vi "Sequence Update.vi"(8 "error in (no error)":errorcluster, 10 "Sequence Record":T2, 11 "Connection Refnum":T1) -> (0 "error out":errorcluster, 3 "Connection Refnum":T1)   [LabVIEW 2011]
uses:
  Sequence Record.ctl
  SI.LIB/ODBC/SQL Controls/Connection Refnum.ctl
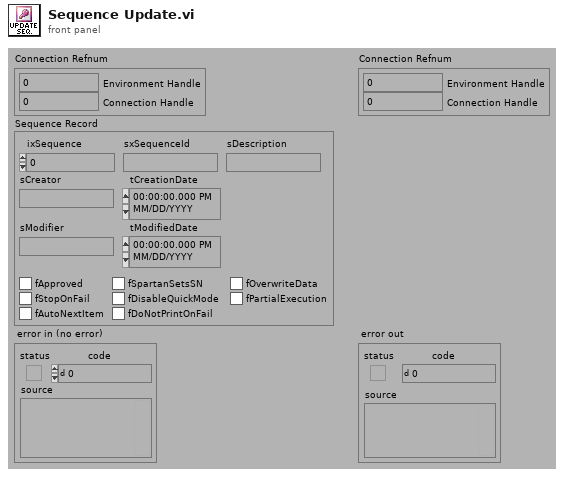
[diagram p1: front panel]
types:
  T1 = typedef "Connection Refnum.ctl" = cluster{"Environment Handle":i32, "Connection Handle":i32}
  T2 = typedef "Sequence Record.ctl" = cluster{"ixSequence":i32, "sxSequenceId":string, "sDescription":string, "sCreator":string, "tCreationDate":timestamp, "sModifier":string, "tModifiedDate":timestamp, "fApproved":bool, "fSpartanSetsSN":bool, "fOverwriteData":bool, "fStopOnFail":bool, "fDisableQuickMode":bool, "fPartialExecution":bool, "fAutoNextItem":bool, "fDoNotPrintOnFail":bool}
  T3 = typedef "Statement Refnum.ctl" = cluster{"Statement Handle":i32, "Parameter Number":u16}
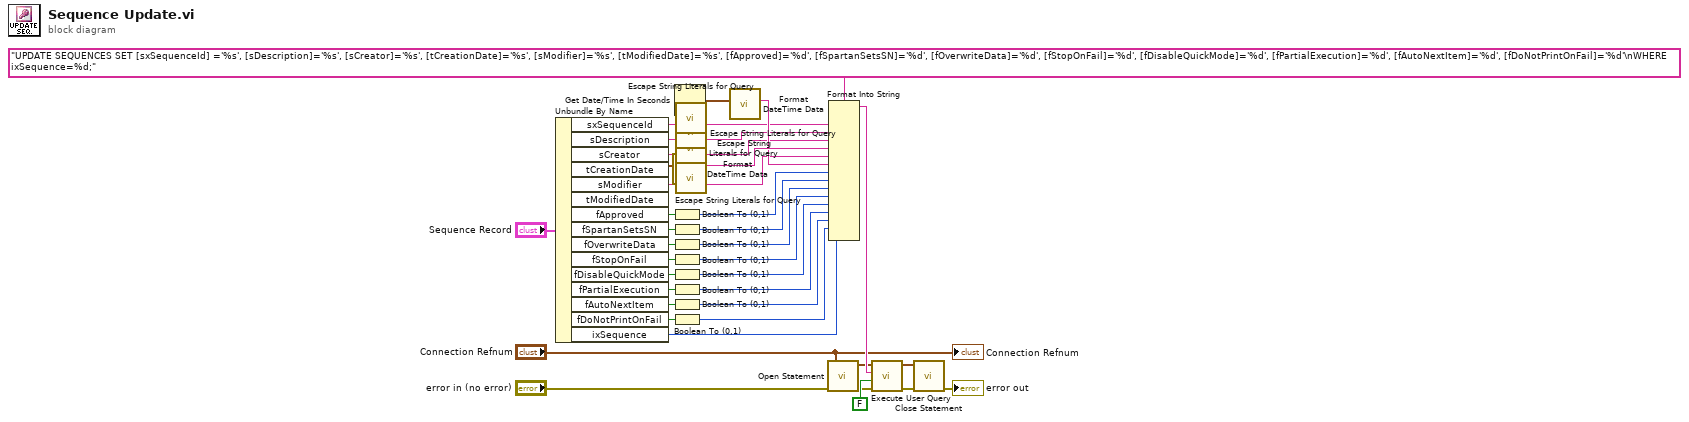
[diagram p0: block diagram]
diagram:
  n1 = Unbundle By Name("Sequence Record") -> ("sxSequenceId"=w11:string, "sDescription"=w9:string, "sCreator"=w8:string, "tCreationDate"=w14:timestamp, "sModifier"=w10:string, "fApproved"=w28:bool, "fSpartanSetsSN"=w27:bool, "fOverwriteData"=w26:bool, "fStopOnFail"=w25:bool, "fDisableQuickMode"=w24:bool, "fPartialExecution"=w23:bool, "fAutoNextItem"=w29:bool, "fDoNotPrintOnFail"=w2:bool, "ixSequence"=w15:i32)  [unwired: 1 out]
  n2 = Boolean To (0,1)(Boolean=w28) -> (0, 1=w22:i16)
  n3 = Boolean To (0,1)(Boolean=w27) -> (0, 1=w21:i16)
  n4 = Boolean To (0,1)(Boolean=w26) -> (0, 1=w20:i16)
  n5 = Boolean To (0,1)(Boolean=w25) -> (0, 1=w19:i16)
  n6 = Boolean To (0,1)(Boolean=w24) -> (0, 1=w18:i16)
  n7 = Boolean To (0,1)(Boolean=w23) -> (0, 1=w17:i16)
  n8 = Boolean To (0,1)(Boolean=w29) -> (0, 1=w16:i16)
  n9 = Boolean To (0,1)(Boolean=w2) -> (0, 1=w1:i16)
  n10 = call "Format DateTime Data.vi"("Timestamp in"=w14) -> ("UTC DB String out"=w13:string)  [unwired: 10 out]
  n11 = Get Date/Time In Seconds() -> (seconds since 1Jan1904=w3:timestamp)
  n12 = call "Escape String Literals for Query.vi"("String"=w11) -> ("escaped String"=w4:string)  [unwired: 1 in, 13 out]
  n13 = call "Escape String Literals for Query.vi"("String"=w9) -> ("escaped String"=w6:string)  [unwired: 1 in, 13 out]
  n14 = call "Escape String Literals for Query.vi"("String"=w8) -> ("escaped String"=w7:string)  [unwired: 1 in, 13 out]
  n15 = call "Escape String Literals for Query.vi"("String"=w10) -> ("escaped String"=w5:string)  [unwired: 1 in, 13 out]
  n16 = call "Format DateTime Data.vi"("Timestamp in"=w3) -> ("UTC DB String out"=w12:string)  [unwired: 10 out]
  n17 = call "Open Statement.vi"("error in (no error)"="error in (no error)", "Connection Refnum"="Connection Refnum") -> ("error out"=w34:errorcluster, "Statement Refnum"=w33:T3)  [unwired: 4 out]
  n18 = Format Into String(format string="UPDATE SEQUENCES SET [sxSequenceId] ='%s', [sDescription]='%s', [sCreator]='%s', [tCreationDate]='%s', [sModifier]='%s', [tModifiedDate]='%s', [fApproved]='%d', [fSpartanSetsSN]='%d', [fOverwriteData]='%d', [fStopOnFail]='%d', [fDisableQuickMode]='%d', [fPartialExecution]='%d', [fAutoNextItem]='%d', [fDoNotPrintOnFail]='%d'\nWHERE ixSequence=%d;" ("User Query"), w4, w6, w7, w13, w5, w12, w22, w21, w20, w19, w18, w17, w16, w1, w15) -> (resulting string=w35:string)  [unwired: 2 in, 1 out]
  n19 = call "Execute User Query.vi"("error in (no error)"=w34, "Return Data? (f)"=FALSE, "User Query"=w35, "Statement Refnum"=w33) -> ("error out"=w38:errorcluster, "Statement Refnum"=w37:T3)  [unwired: 2 out]
  n20 = call "Close Statement.vi"("error in (no error)"=w38, "Statement Refnum"=w37) -> ("error out"=→"error out":errorcluster)  [unwired: 5 out]
  "Connection Refnum" <- "Connection Refnum"
